vi "save to drive.vi"(8 "error in (no error)":errorcluster, 11 "DAQCascade512II in":refnum<class "DAQCascade512II.lvclass">) -> (0 "error out":errorcluster, 3 "DAQCascade512II out":refnum<class "DAQCascade512II.lvclass">)   [LabVIEW 2012, in "DAQCascade512II.lvclass"]
uses:
  DAQCascade512II.lvclass
  DAQCascade512II.lvclass/DAQCascade512II.ctl
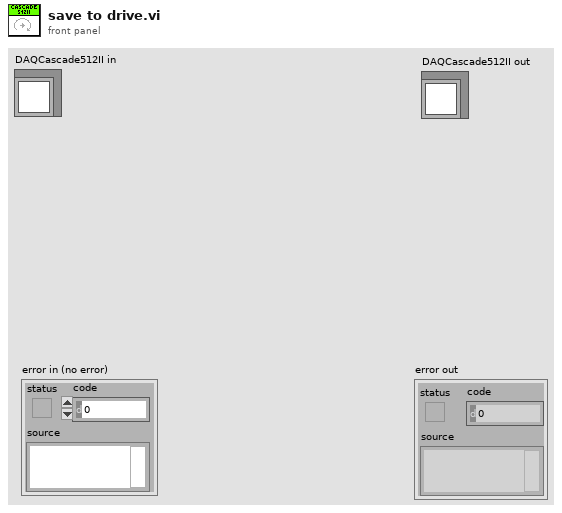
[diagram p1: front panel]
types:
  T1 = typedef "DAQCascade512II.lvclass/no. of frames.ctl" = u32
  T2 = typedef "IMAQ Image.ctl" = refnum<image>
  T3 = cluster{"Rows Per Strip":i32, "Photometric":i32, "Compression Type":i32}
  T4 = cluster{"Array uint 16":u16[][], "setting.File Path":path}
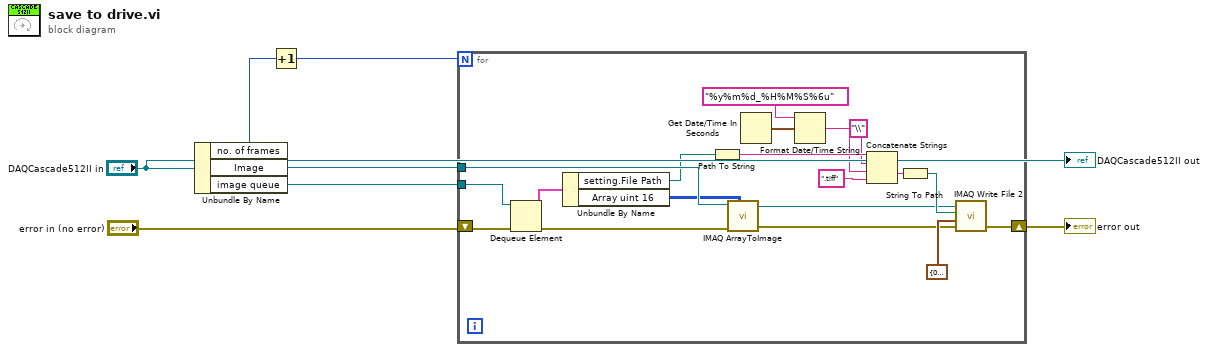
[diagram p0: block diagram]
diagram:
  n1 = Unbundle By Name("DAQCascade512II in") -> ("no. of frames"=w1:T1, "Image"=w3:T2, "image queue"=w5:refnum<queue>)
  n2 = Increment(x=w1) -> (x+1=w2:T1)
  n3 = for {
    N: w2 -> [_]
    tunnel: w5 -> [w16]
    tunnel: w3 -> [w13]
    shift-right: [w17] -> w7
    shift-left: "error in (no error)" -> [w15]
    n4 = Dequeue Element(queue=w16, error in (no error)=w15) -> (element=w14:T4, error out=w11:errorcluster)  [unwired: 1 in, 2 out]
    n5 = Unbundle By Name(w14) -> ("setting.File Path"=w10:path, "Array uint 16"=w12:u16[][])
    n6 = Path To String(path=w10) -> (string=w23:string)
    n7 = call "IMAQ ArrayToImage"("Image Pixels (U16)"=w12, "error in (no error)"=w11, "Image"=w13) -> ("error out"=w8:errorcluster, "Image Out"=w9:T2)  [unwired: 7 in]
    n8 = Get Date/Time In Seconds() -> (seconds since 1Jan1904=w24:timestamp)
    n9 = Format Date/Time String(time format string (%c)="%y%m%d_%H%M%S%6u", seconds (now)=w24) -> (date/time string=w21:string)  [unwired: 1 in]
    n10 = Concatenate Strings(w23, "\\" ("string"), w21, ".tiff" ("string")) -> (w19:string)
    n11 = String To Path(string=w19) -> (path=w18:path)
    n12 = call-poly "IMAQ Write File 2"("error in (no error)"=w8, "TIFF Options"=T3 {"Rows Per Strip"=0, "Photometric"=1, "Compression Type"=0}, "File Path"=w18, "Image"=w9) -> ("error out"=w17:errorcluster)  [unwired: 6 in, 1 out]
  }
  "error out" <- w7
  "DAQCascade512II out" <- "DAQCascade512II in"
